vi "Scan_FileList.vi"(11 "Data Feed":string) -> (0 "Downloaded bytes":i32, 2 "state out":string, 3 "Sorted Files":string[][](array[string]))   [LabVIEW 2020]
uses:
  DataCluster.ctl
  bf192da2-a038-4d3f-ab57-7c4c3700bcdc.vi
  <vilib>/Array/Sort 2D Array - Pop Stack.vi
  <vilib>/Array/Sort 2D Array - Push Stack.vi
panel:
  in  "DataCluster":T1
  out "substring before match":string
  out "Array":string[][](array[string])
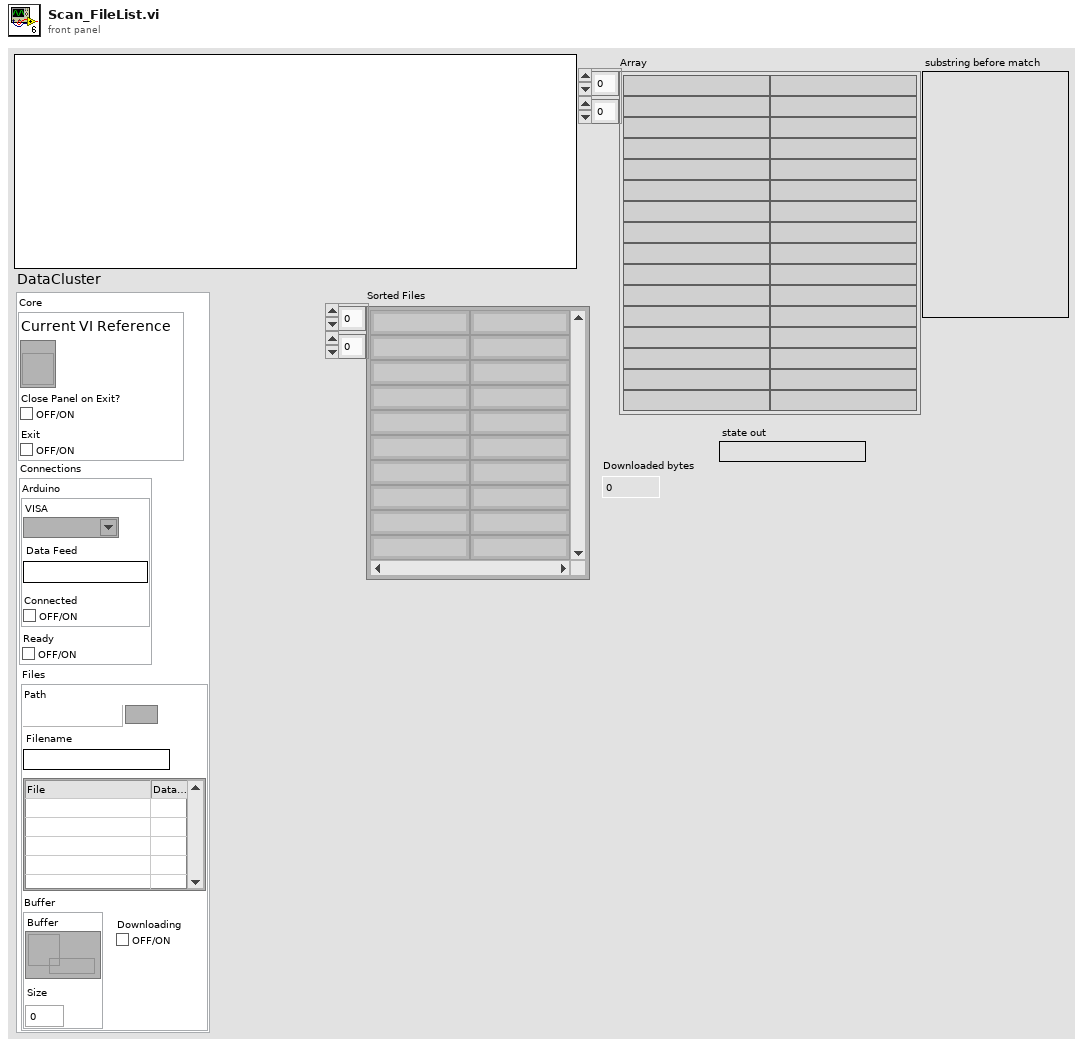
[diagram p1: front panel]
types:
  T1 = typedef "DataCluster.ctl" = cluster{"Core":cluster{"Current VI Reference":refnum<vi>, "Close Panel on Exit?":bool, "Exit":bool}, "Connections":cluster{"Arduino":cluster{"VISA":refnum<visa-resource-name>, "Data Feed":string, "Connected":bool}, "Ready":bool}, "Files":cluster{"Path":path, "Filename":string, "File List":i32, "Buffer":cluster{"Buffer":refnum<queue>, "Size":i32}, "Downloading":bool}}
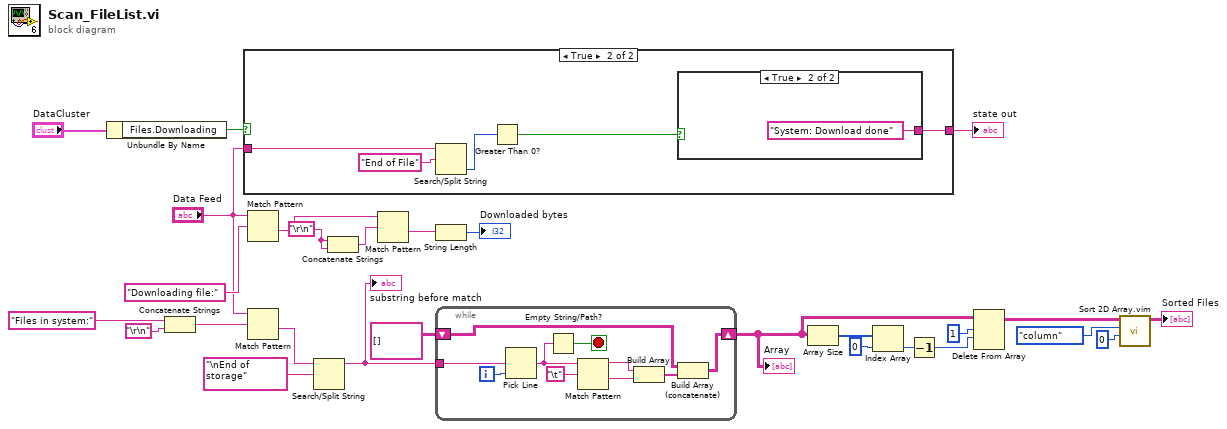
[diagram p0: block diagram]
diagram:
  w10 = "\r\n"
  n1 = Unbundle By Name("DataCluster") -> ("Files.Downloading"=w3:bool)
  n2 = Concatenate Strings("Files in system:" ("search string/char (-)"), "\r\n") -> (w26:string)
  n3 = case shown="True" w3 {
    tunnel: "Data Feed" -> [_ w32]
    tunnel: [_ w28] -> w1
    frame False {
    }
    frame True {
      n4 = Search/Split String(string=w32, search string/char (-)="End of File") -> (offset of match=w30:i32)  [unwired: 1 in, 2 out]
      n5 = Greater Than 0?(x=w30) -> (x > 0?=w29:bool)
      n6 = case shown="True" w29 {
        tunnel: [_ "System: Download done"] -> w28
        frame False {
        }
        frame True {
        }
      }
    }
  }
  "state out" <- w1
  n7 = Match Pattern(string="Data Feed", regular expression="Downloading file:") -> (after substring=w8:string)  [unwired: 1 in, 3 out]
  n8 = Match Pattern(string="Data Feed", regular expression=w26) -> (after substring=w25:string)  [unwired: 1 in, 3 out]
  n9 = Search/Split String(string=w25, search string/char (-)="\nEnd of storage") -> (substring before match=w23:string)  [unwired: 1 in, 2 out]
  "substring before match" <- w23
  n10 = Concatenate Strings(w10, w10) -> (w7:string)
  n11 = Match Pattern(string=w8, regular expression=w7) -> (after substring=w6:string)  [unwired: 1 in, 3 out]
  n12 = String Length(string=w6) -> (length=→"Downloaded bytes":i32)
  n13 = while {
    tunnel: w23 -> [w43]
    shift-right: [w36] -> w15
    shift-left: string[][] [] -> [w35]
    i -> [w42]
    stop <- w41 stop-if-true
    n14 = Pick Line(multi-line string=w43, line index=w42) -> (output string=w40:string)  [unwired: 1 in]
    n15 = Empty String/Path?(string/path=w40) -> (empty?=w41:bool)
    n16 = Match Pattern(string=w40, regular expression="\t") -> (before substring=w39:string, after substring=w38:string)  [unwired: 1 in, 2 out]
    n17 = Build Array(w39, w38) -> (w37:string[])
    n18 = Build Array (concatenate)(w35, w37) -> (w36:string[][])
  }
  "Array" <- w15
  n19 = Array Size(array=w15) -> (size(s)=w20:i32[])
  n20 = Index Array(array=w20, index=0) -> (element=w18:i32)
  n21 = Decrement(x=w18) -> (x-1=w16:i32)
  n22 = Delete From Array(array=w15, length=1, index (row)=w16) -> (array with subset deleted=w11:string[][])  [unwired: 1 in, 1 out]
  n23 = call "Sort 2D Array.vim"("index"=0, "dimension to index (column)"=enum16{"column", "row"}."column", "2D array"=w11) -> ("sorted 2D array"=→"Sorted Files":string[][])  [unwired: 7 in, 1 out]
